vi "CfgManager.Text Partial Found Test Launcher.vi"() -> ()   [LabVIEW 2013]
uses:
  <vilib>/LabVIEW Open Source Project/Unicity/Delimiter/Delimiters List.ctl
  source/Manager.Text/ConfigManager.Text.lvclass
  source/Manager.Text/ConfigManager.Text.lvclass/ConfigManager.Text.ctl
  <vilib>/LabVIEW Open Source Project/Unicity/Delimiter/Delimiter.lvclass
  source/Manager/ConfigManager.lvclass
panel:
  out "any found?":bool
  out "all found?":bool
  out "default pump config":variant
  out "default config":path
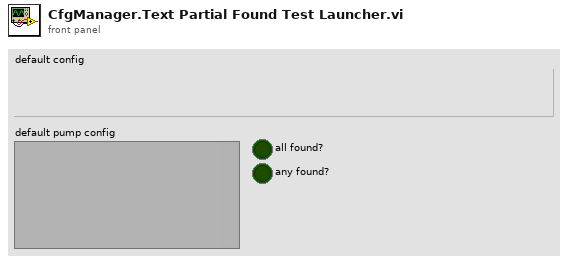
[diagram p1: front panel]
types:
  T1 = cluster{"String":string, "Numeric":dbl, "Boolean":bool}
  T2 = typedef "Delimiter.lvclass/Delimiters List.ctl" = enum16{"Default", "dot (.)", "colon (:)", "double-colon (::)", "semi-colon (;)", "underscore (_)", "double underscore (__)", "dash (-)", "double dash (--)", "backslash (\\)", "vertical bar (|)", "forward slash (/)", "chevron (>)", "double-chevron (>>)", "arrow (->)", "comma (,)", "arobas (@)", "ampersand (&)", "other"}
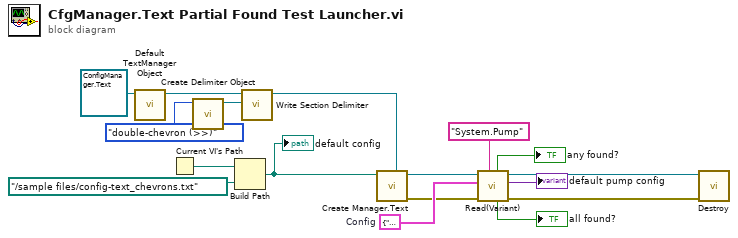
[diagram p0: block diagram]
diagram:
  w9 = T1 {"String"="", "Numeric"=0.0, "Boolean"=FALSE}  # Config
  n1 = call-dynamic "Default TextManager Object.vi"("CfgManager.Text in"=refnum<class "ConfigManager.Text.lvclass"> refnum) -> ("CfgManager.Text out"=w15:refnum<class "ConfigManager.Text.lvclass">)  [unwired: 10 in]
  n2 = Current VI's Path() -> (path=w6:path)
  n3 = call <vilib>:"Create Delimiter Object.vi"("Delimiter"=Delimiters_List."double-chevron (>>)") -> ("Delimiter"=w16:refnum<class "Delimiter.lvclass">)  [unwired: 10 in]
  n4 = Build Path(base path=w6, name or relative path=path "../sample files/config-text_chevrons.txt" ("filepath 2")) -> (appended path=w4:path)
  "default config" <- w4
  n5 = call "Write Section Delimiter.vi"("Section Delimiter"=w16, "ConfigManager.Text in"=w15) -> ("ConfigManager.Text out"=w14:refnum<class "ConfigManager.Text.lvclass">)  [unwired: 9 in]
  n6 = call "Create Manager.Text.vi"("ConfigManager.Text"=w14, "filepath"=w4) -> ("error out"=w2:errorcluster, "ConfigManager.Text out"=w12:refnum<class "ConfigManager.Text.lvclass">)  [unwired: 7 in, 1 out]
  n7 = call "Read(Variant).vi"("Qualified Name"="System.Pump", "error in (no error)"=w2, "Type"=w9, "ConfigManager in"=w12) -> ("error out"=w1:errorcluster, "value"=→"default pump config":variant, "ConfigManager out"=w7:refnum<class "ConfigManager.Text.lvclass">, "all found?"=→"all found?":bool, "any found?"=→"any found?":bool)  [unwired: 3 in]
  n8 = call-dynamic "Destroy.vi"("error in (no error)"=w1, "ConfigManager.Text in"=w7) -> ()  [unwired: 8 in, 2 out]
